vi "Get AeroScript Status.vi"(8 "error in (no error)":errorcluster, 10 "taskId":T1(ring)=enum."T01", 11 "Gantry in":refnum<class "Gantry.lvclass">) -> (0 "error out":errorcluster, 2 "State":i32, 3 "Gantry out":refnum<class "Gantry.lvclass">)   [LabVIEW 2026, in "Gantry.lvclass"]
uses:
  Gantry.lvclass
  C:/Users/User/Desktop/pixel-gantry-control/Gantry/A3200/Bin/Aerotech.A3200.LabVIEW.dll
  A3200/Bin/Aerotech.A3200.LabVIEW.dll
  C:/Users/User/Desktop/pixel-gantry-control/Gantry/A3200/Bin/Aerotech.A3200.dll
  A3200/Bin/Aerotech.A3200.dll
  <instrlib>/Aerotech Automation1/Aerotech Automation1.lvlib
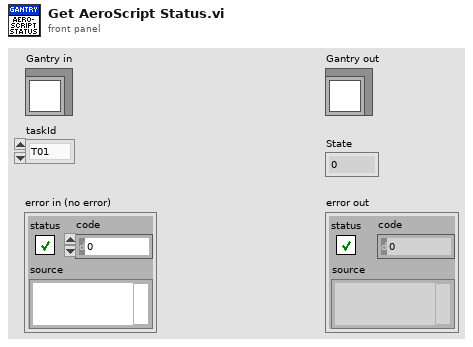
[diagram p1: front panel]
types:
  T1 = enum16{"TLibrary", "T01", "T02", "T03", "T04", "T05", "T06", "T07", "T08", "T09", "T10", "T11", "T12", "T13", "T14", "T15", "T16", "T17", "T18", "T19", "T20", "T21", "T22", "T23", "T24", "T25", "T26", "T27", "T28", "T29", "T30", "T31"}
  T2 = typedef "Virtual Modes.ctl" = enum16{"Nonvirtual", "Virtual"}
  T3 = typedef "Aerotech Automation1.lvlib/Task Status Cluster.ctl" = cluster{"TaskState":T4, "TaskMode":i32, "AeroScriptSourceFileName":string, "CompiledAeroScriptFileName":string, "ManualFeedrateOverride":dbl, "Warning Number":i32, "Warning Message":string, "Error Number":i32, "Error Message":string}
  T4 = typedef "Aerotech Automation1.lvlib/Task State.ctl" = enum16{"Unavailable", "Inactive", "Idle", "ProgramReady", "ProgramRunning", "ProgramFeedhold", "ProgramPaused", "ProgramComplete", "Error", "Queue"}
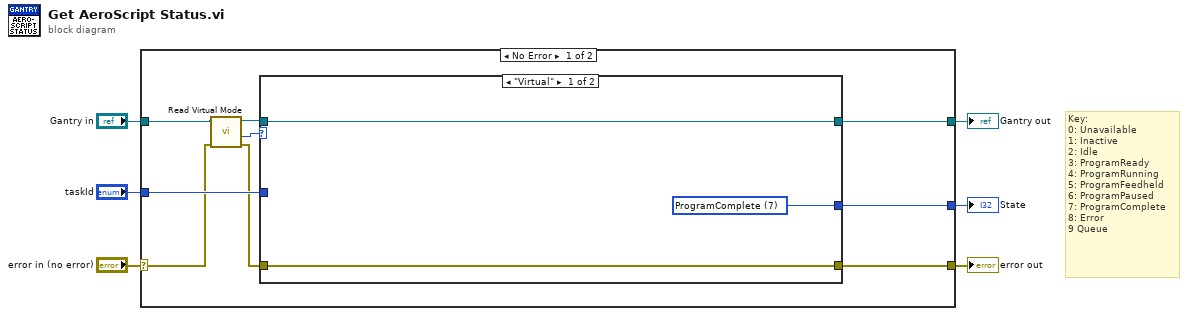
[diagram p0: block diagram]
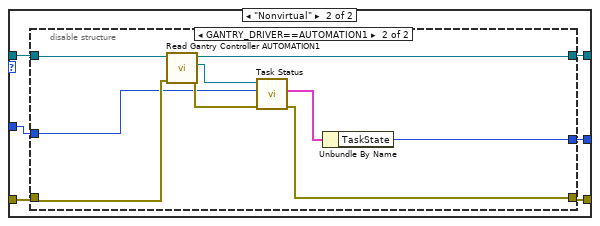
[diagram p2: hidden frame]
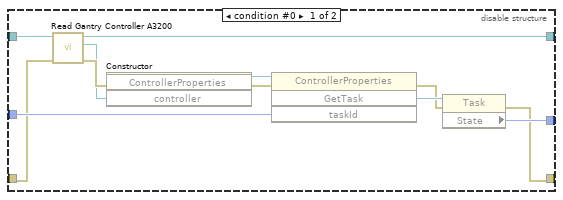
[diagram p3: hidden frame]
diagram:
  # "Key:\n0: Unavailable\n1: Inactive\n2: Idle\n3: ProgramReady\n4: ProgramRunning\n5: ProgramFeedheld\n6: ProgramPaused\n7: ProgramComplete\n8: Error\n9 Queue"
  n1 = case shown="No Error" "error in (no error)" {
    selector: "error in (no error)" -> [w8 w47]
    tunnel: [w12 w47] -> w5
    tunnel: [w15 w46] -> w3
    tunnel: "Gantry in" -> [w11 w46]
    tunnel: [w14 _] -> w2
    tunnel: "taskId" -> [w13 _]
    frame No Error {
      n2 = call-dynamic "Read Virtual Mode.vi"("error in (no error)"=w8, "Gantry in"=w11) -> ("error out"=w7:errorcluster, "Virtual Mode"=w9:T2, "Gantry out"=w10:refnum<class "Gantry.lvclass">)  [unwired: 6 in, 1 out]
      n3 = case shown="\"Virtual\"" w9 {
        tunnel: w7 -> [w16 w19]
        tunnel: [w17 w20] -> w15
        tunnel: [w16 w22] -> w12
        tunnel: w10 -> [w17 w21]
        tunnel: w13 -> [_ w24]
        tunnel: [w18 w23] -> w14
        frame "Virtual" {
          w18 = 7 items=["Unavailable", "Inactive", "Idle", "ProgramReady", "ProgramRunning", "ProgramFeedheld", "ProgramPaused", "ProgramComplete", "Error", "Queue"] ("State")
        }
        frame "Nonvirtual" {
          n4 = disable-structure shown="GANTRY_DRIVER==AUTOMATION1" {
            disable-tunnel: w24 -> [w34 w37]
            disable-tunnel: [w31 w39] -> w23
            disable-tunnel: [w30 w40] -> w22
            disable-tunnel: w21 -> [w29 w42]
            disable-tunnel: [w28 w38] -> w20
            disable-tunnel: w19 -> [w27 w41]
            frame condition #0 {
              n5 = call "Read Gantry Controller A3200.vi"("error in (no error)"=w27, "Gantry in"=w29) -> ("error out"=w26:errorcluster, "A3200 controller out"=w25:refnum<k24>, "Gantry out"=w28:refnum<class "Gantry.lvclass">)  [unwired: 7 in]
              n6 = constructor class="ControllerProperties"(error in=w26, "controller"=w25) -> (reference out=w35:refnum<k24>, error out=w36:errorcluster)  [unwired: 2 in, 2 out]
              n7 = invoke class="ControllerProperties" method="GetTask"(reference=w35, error in=w36, "taskId"=w34) -> (error out=w32:errorcluster, "GetTask"=w33:refnum<k24>)  [unwired: 1 in, 2 out]
              n8 = property class="Task"(reference=w33, error in=w32) -> (error out=w30:errorcluster, "State"=w31:i32)  [unwired: 1 out]
            }
            frame condition #1 (active) {
              n9 = call "Read Gantry Controller AUTOMATION1.vi"("error in (no error)"=w41, "Gantry in"=w42) -> ("error out"=w44:errorcluster, "Controller AUTOMATION1"=w45:refnum<k24>, "Gantry out"=w38:refnum<class "Gantry.lvclass">)  [unwired: 7 in]
              n10 = call <instrlib>:"Task Status.vi"("error in (no error)"=w44, "Task Index"=w37, "Controller Refnum"=w45) -> ("error out"=w40:errorcluster, "Task Status Cluster"=w43:T3)  [unwired: 6 in, 1 out]
              n11 = Unbundle By Name(w43) -> ("TaskState"=w39:T4)
            }
          }
        }
      }
    }
    frame Error {
    }
  }
  "error out" <- w5
  "Gantry out" <- w3
  "State" <- w2
